vi "APXGauge191119.vi"() -> ()   [LabVIEW 2015]
uses:
  <vilib>/Instr/_visa.llb/VISA Configure Serial Port (Instr).vi
  <userlib>/caLab/Private/Get_PV-1D.vi
  <userlib>/caLab/Private/Put_DBL-1D_PV-1D.vi
  <vilib>/Utility/config.llb/Read Key (String).vi
  <vilib>/Utility/config.llb/NI_LVConfig.lvlib
  <vilib>/Utility/config.llb/Read Key (Path).vi
panel:
  out "APX:SP_SES100":bool
  out "Numeric 3":i32
  in  "stop 2":bool
  out "Numeric 2":i32
  in  "stop":bool
  out "BL132:132WRG1":dbl
  out "SP HIGH":string
  out "SP LOW":string
  out "BL132:SP_BL132":bool
  out "VISA resource name":refnum<visa-resource-name>="COM26"
  out "COM TN908A":refnum<visa-resource-name>="COM10"
  out "APX:GAS":dbl format="%_3f"
  out "APX:AUX":dbl format="%_3f"
  out "COM MAXIGAUGE":refnum<visa-resource-name>
  out "Status":bool
  out "APX:SP_F":bool
  out "APX:SP_E":bool
  out "APX_SP_D":bool
  out "APX:SP_C":bool
  out "APX:SP_B":bool
  out "APX:SP_A":bool
  out "Cycle":i32
  out "APX:HPC001":dbl format="%.6f"
  out "APX:AP2":dbl format="%#_3e"
  out "APX:AP1":dbl format="%#_4g"
  out "APX:PREP":dbl format="%#_3g"
  out "APX:HPC":dbl format="%#_3g"
  out "APX:HPC100":dbl format="%.5g"
  out "APX:SEN6_OFF":bool
  out "APX:SEN6_ON":bool
  out "APX:SEN5_OFF":bool
  out "APX:SEN5_ON":bool
  out "APX:SEN4_OFF":bool
  out "APX:SEN4_ON":bool
  out "APX:SEN3_OFF":bool
  out "APX:SEN3_ON":bool
  out "APX:SEN2_OFF":bool
  out "APX:SEN2_ON":bool
  out "APX:SEN1_OFF":bool
  out "APX:SEN1_ON":bool
  in  "STOP":bool
  # "APX Gauges"
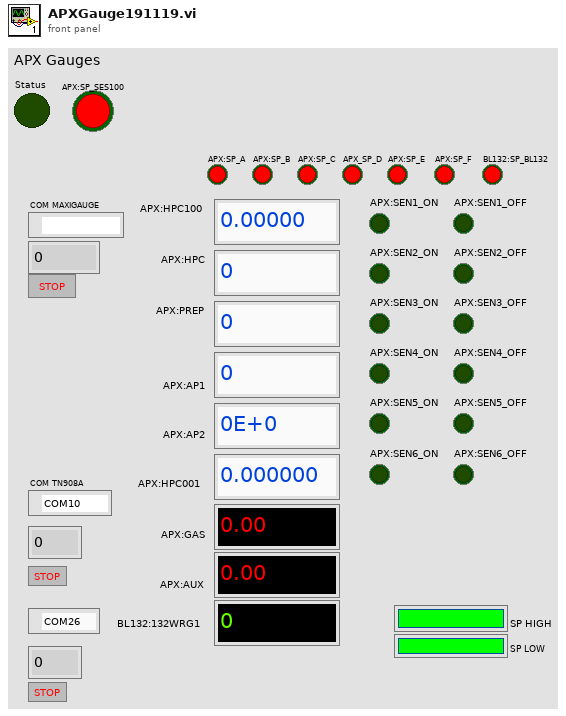
[diagram p1: front panel]
types:
  T1 = typedef "NI_LVConfig.lvlib/Config Data RefNum.ctl" = refnum<k1>
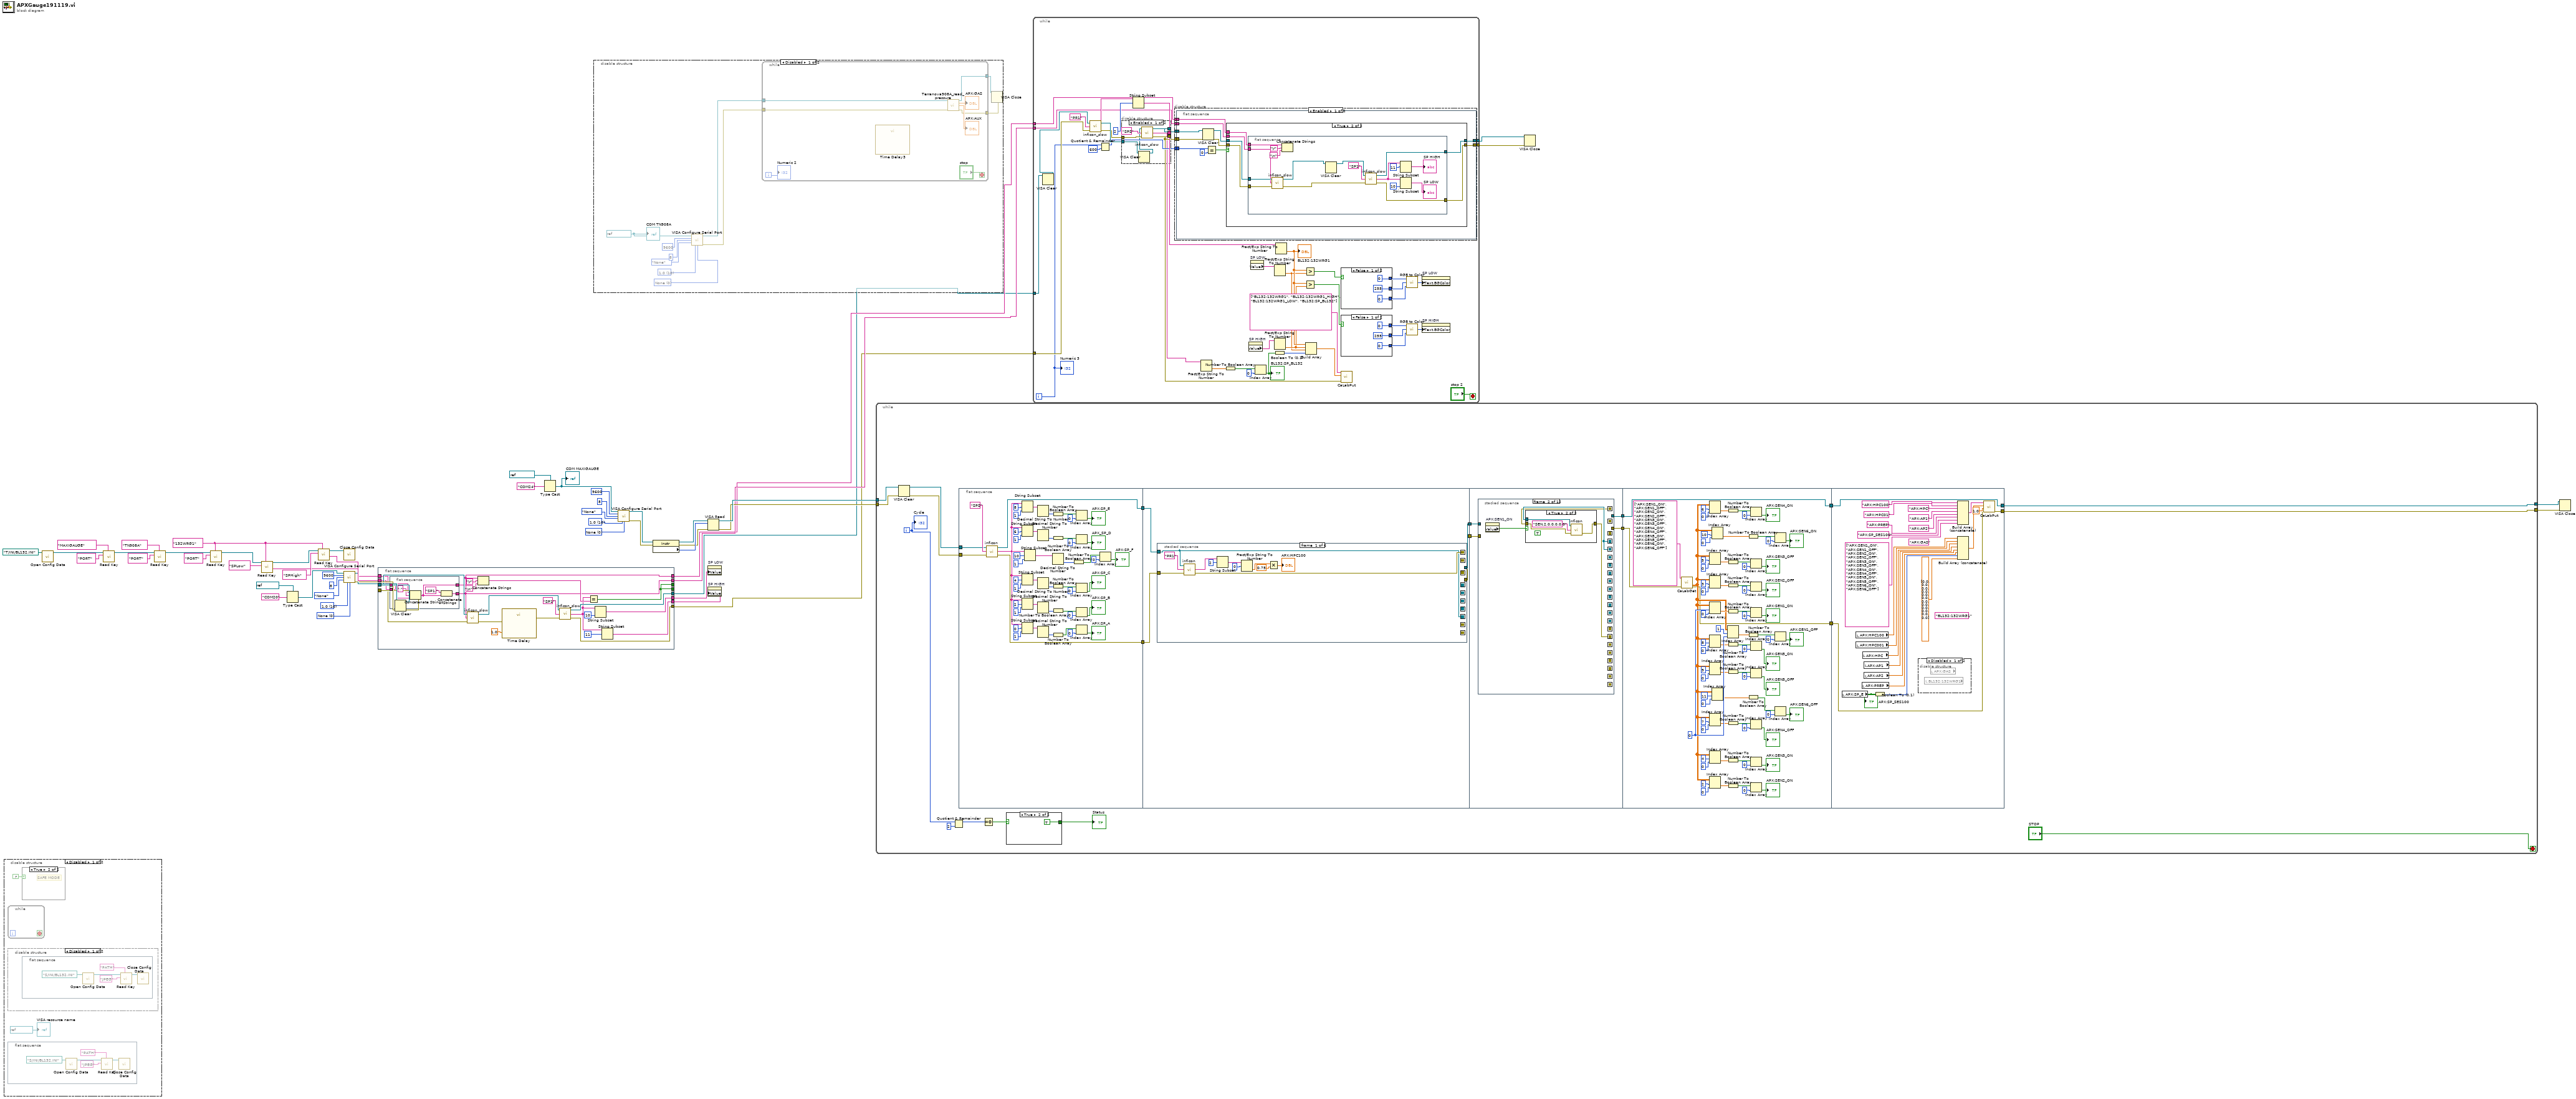
[diagram p0: block diagram]
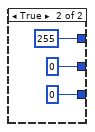
[diagram p6: hidden frame]
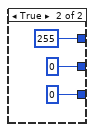
[diagram p7: hidden frame]
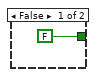
[diagram p11: hidden frame]
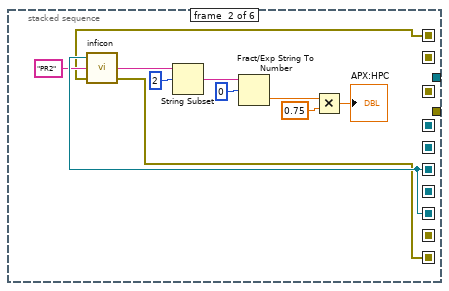
[diagram p12: hidden frame]
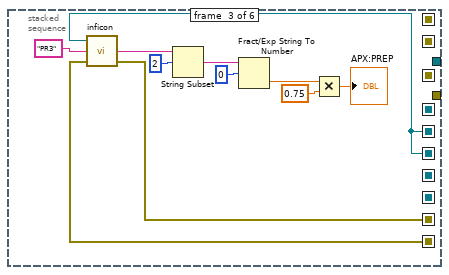
[diagram p13: hidden frame]
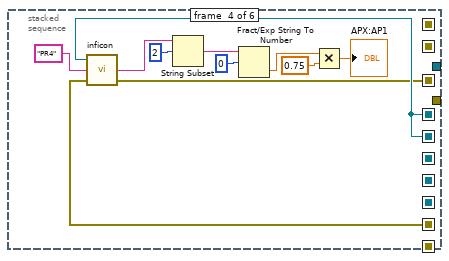
[diagram p14: hidden frame]
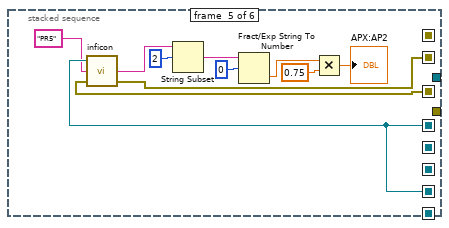
[diagram p15: hidden frame]
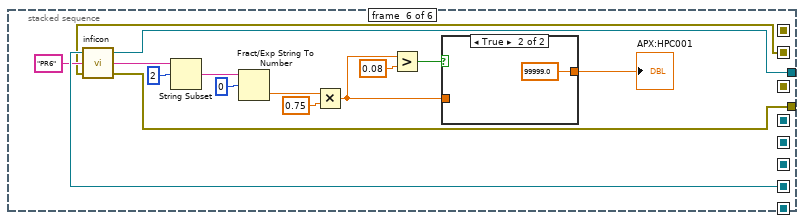
[diagram p16: hidden frame]
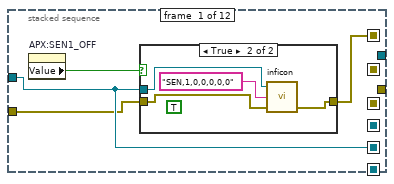
[diagram p18: hidden frame]
diagram:
  w23 = "132WRG1" ("y")
  w33 = u16 10 items=["1.0"=10, "1.5"=15, "2.0"=20] ("stop bits (10: 1 bit)")
  w34 = u16 0 items=["None", "XON/XOFF", "RTS/CTS", "XON/XOFF & RTS/CTS", "DTR/DSR", "XON/XOFF & DTR/DSR"] ("flow control (0:none)")
  w50 = u16 10 items=["1.0"=10, "1.5"=15, "2.0"=20] ("stop bits (10: 1 bit)")
  w51 = u16 0 items=["None", "XON/XOFF", "RTS/CTS", "XON/XOFF & RTS/CTS", "DTR/DSR", "XON/XOFF & DTR/DSR"] ("flow control (0:none)")
  n1 = disable-structure shown="Disabled" {
    frame Disabled {
      n2 = while {
        stop <- _ stop-if-true
      }
      n3 = disable-structure shown="Disabled" {
        frame Disabled {
          n4 = flat-sequence {
            frame #0 {
              n5 = call <vilib>:"Open Config Data.vi"("configuration file path"=path "S:/INI/BL132.INI") -> ("refnum"=w58:T1)  [unwired: 8 in, 2 out]
              n6 = call-poly <vilib>:"Read Key.vi"("section"="PATH" ("key"), "key"="JPEG" ("section"), "refnum"=w58) -> ("value"=w57:path, "refnum out"=w62:T1)  [unwired: 5 in, 2 out]
              n7 = call <vilib>:"Close Config Data.vi"("refnum"=w62) -> ()  [unwired: 9 in, 2 out]
            }
          }
        }
        frame Enabled {
        }
      }
      n8 = flat-sequence {
        frame #0 {
          n9 = call <vilib>:"Open Config Data.vi"("configuration file path"=path "S:/INI/BL132.INI") -> ("refnum"=w63:T1)  [unwired: 8 in, 2 out]
          n10 = call-poly <vilib>:"Read Key.vi"("section"="PATH" ("key"), "key"="JPEG" ("section"), "refnum"=w63) -> ("refnum out"=w67:T1)  [unwired: 5 in, 3 out]
          n11 = call <vilib>:"Close Config Data.vi"("refnum"=w67) -> ()  [unwired: 9 in, 2 out]
        }
      }
      n12 = case shown="True" FALSE {
        frame False {
        }
        frame True {
          # "SAFE MODE"
        }
      }
      "VISA resource name" <- refnum<visa-resource-name> "COM1" ("VISA resource name")
    }
    frame Enabled {
    }
  }
  n13 = call <vilib>:"Open Config Data.vi"("configuration file path"=path "T:/INI/BL132.INI") -> ("refnum"=w12:T1)  [unwired: 8 in, 2 out]
  n14 = call-poly <vilib>:"Read Key.vi"("section"="MAXIGAUGE" ("y"), "key"="PORT" ("y"), "refnum"=w12) -> ("refnum out"=w13:T1)  [unwired: 5 in, 3 out]
  n15 = call-poly <vilib>:"Read Key.vi"("section"="TN908A" ("y"), "key"="PORT" ("y"), "refnum"=w13) -> ("refnum out"=w11:T1)  [unwired: 5 in, 3 out]
  n16 = call-poly <vilib>:"Read Key.vi"("section"=w23, "key"="PORT" ("y"), "refnum"=w11) -> ("refnum out"=w21:T1)  [unwired: 5 in, 3 out]
  n17 = call-poly <vilib>:"Read Key.vi"("section"=w23, "key"="SPLow" ("y"), "refnum"=w21) -> ("value"=w25:string, "refnum out"=w29:T1)  [unwired: 5 in, 2 out]
  n18 = Type Cast(type=refnum<visa-resource-name> "COM1" ("VISA resource name"), x="COM20") -> (*(type *) &x=w31:refnum<visa-resource-name>)
  n19 = call-poly <vilib>:"Read Key.vi"("section"=w23, "key"="SPHigh" ("y"), "refnum"=w29) -> ("value"=w24:string, "refnum out"=w30:T1)  [unwired: 5 in, 2 out]
  n20 = call <vilib>:"Close Config Data.vi"("refnum"=w30) -> ()  [unwired: 9 in, 2 out]
  n21 = call-poly "VISA Configure Serial Port"("VISA resource name"=w31, "baud rate (9600)"=u32 9600, "data bits (8)"=u16 8, "parity (0:none)"=enum16{"None", "Odd", "Even", "Mark", "Space"}."None", "stop bits (10: 1 bit)"=w33, "flow control (0:none)"=w34) -> ("VISA resource name out"=w10:refnum<visa-resource-name>, "error out"=w8:errorcluster)  [unwired: 8 in]
  n22 = flat-sequence {
    tunnel: w9 -> [w86]
    tunnel: w7 -> [w84]
    tunnel: w25 -> [w69]
    tunnel: w24 -> [w68]
    tunnel: [w88] -> w4
    tunnel: [w87] -> w3
    tunnel: [w72] -> _
    tunnel: [w74] -> w18
    tunnel: [w73] -> w19
    tunnel: [w72] -> _
    tunnel: [w71] -> w6
    tunnel: [w70] -> w5
    frame #0 {
      n23 = flat-sequence {
        tunnel: [w92] -> w71
        tunnel: [w93] -> w70
        tunnel: w69 -> [w91]
        tunnel: w68 -> [w90]
        frame #0 {
          n24 = Concatenate Strings(w91, "," ("string to write"), w90) -> (w93:string)
          n25 = Concatenate Strings("SP1," ("string to write"), w93) -> (w92:string)
        }
      }
      n26 = call "inficon_slow.vi"("error out"=w84, "string to write"=w71, "VISA resource name"=w86) -> ("error out 2"=w82:errorcluster, "VISA resource name 2"=w85:refnum<visa-resource-name>)  [unwired: 1 out]
      n27 = Concatenate Strings(w70, "\r", "\n") -> (w80:string)
      n28 = call "Time Delay"("error in (no error)"=w82, "Delay Time (s)"=1.0) -> ("error out"=w83:errorcluster)  [unwired: 9 in]
      n29 = call "inficon_slow.vi"("error out"=w83, "string to write"="SP1", "VISA resource name"=w85) -> ("error out 2"=w87:errorcluster, "read buffer 2"=w76:string, "VISA resource name 2"=w88:refnum<visa-resource-name>)
      n30 = Equal?(x=w76, y=w80) -> (x = y?=w72:bool)
      n31 = String Subset(string=w76, length (rest)=10 ("length (rest)")) -> (substring=w73:string)  [unwired: 1 in]
      n32 = String Subset(string=w76, offset (0)=11) -> (substring=w74:string)  [unwired: 1 in]
    }
  }
  n33 = VISA Clear(VISA resource name=w10, error in (no error)=w8) -> (VISA resource name out=w9:refnum<visa-resource-name>, error out=w7:errorcluster)
  n34 = Type Cast(type=refnum<visa-resource-name> "COM24" ("VISA resource name"), x="COM24") -> (*(type *) &x=w48:refnum<visa-resource-name>)
  "COM MAXIGAUGE" <- w48
  n35 = disable-structure shown="Disabled" {
    frame Disabled {
      w100 = u16 10 items=["1.0"=10, "1.5"=15, "2.0"=20] ("stop bits (10: 1 bit)")
      w101 = u16 0 items=["None", "XON/XOFF", "RTS/CTS", "XON/XOFF & RTS/CTS", "DTR/DSR", "XON/XOFF & DTR/DSR"] ("flow control (0:none)")
      w105 = refnum<visa-resource-name> "COM10" ("VISA resource name")
      n36 = call-poly "VISA Configure Serial Port"("VISA resource name"=w105, "baud rate (9600)"=u32 9600, "data bits (8)"=u16 8, "parity (0:none)"=enum16{"None", "Odd", "Even", "Mark", "Space"}."None", "stop bits (10: 1 bit)"=w100, "flow control (0:none)"=w101) -> ("VISA resource name out"=w99:refnum<visa-resource-name>, "error out"=w98:errorcluster)  [unwired: 8 in]
      n37 = while {
        tunnel: w99 -> [w111]
        tunnel: w98 -> [w110]
        tunnel: [w109] -> w97
        tunnel: [w108] -> w96
        i -> [w106]
        stop <- "stop" stop-if-true
        n38 = call "Time Delay3"() -> ()  [unwired: 11 in, 1 out]
        n39 = call "Terranova908A_read_pressure.vi"("VISA resource name"=w111, "error in (no error)"=w110) -> ("VISA resource name out"=w109:refnum<visa-resource-name>, "pressure"=→"APX:GAS":dbl, "pressure 2"=→"APX:AUX":dbl, "error out"=w108:errorcluster)  [unwired: 9 in, 1 out]
        "Numeric 2" <- w106
      }
      n40 = VISA Close(VISA resource name=w97, error in (no error)=w96) -> ()  [unwired: 1 out]
      "COM TN908A" <- w105
    }
    frame Enabled {
    }
  }
  n41 = call-poly "VISA Configure Serial Port"("VISA resource name"=w48, "baud rate (9600)"=u32 9600, "data bits (8)"=u16 8, "parity (0:none)"=enum16{"None", "Odd", "Even", "Mark", "Space"}."None", "stop bits (10: 1 bit)"=w50, "flow control (0:none)"=w51) -> ("VISA resource name out"=w45:refnum<visa-resource-name>, "error out"=w38:errorcluster)  [unwired: 8 in]
  n42 = property class="Instr"(reference=w45, error in=w38) -> (reference out=w46:refnum<visa-resource-name>, error out=w39:errorcluster, "Serial Settings:Number of Bytes at Serial Port"=w43:u32)
  n43 = VISA Read(VISA resource name=w46, byte count=w43, error in (no error)=w39) -> (VISA resource name out=w44:refnum<visa-resource-name>, error out=w40:errorcluster)  [unwired: 2 out]
  n44 = property on="SP LOW" class="Str"("Value"=w19) -> ()  [unwired: 2 in, 2 out]
  n45 = property on="SP HIGH" class="Str"("Value"=w18) -> ()  [unwired: 2 in, 2 out]
  n46 = while {
    tunnel: [w127] -> w41
    tunnel: w44 -> [w122]
    tunnel: [w130] -> w42
    tunnel: w40 -> [w120]
    i -> [w114]
    stop <- "STOP" stop-if-true
    n47 = VISA Clear(VISA resource name=w122, error in (no error)=w120) -> (VISA resource name out=w121:refnum<visa-resource-name>, error out=w119:errorcluster)
    n48 = Quotient & Remainder(x=w114, y=2) -> (x-y*floor(x/y)=w117:i32)  [unwired: 1 out]
    n49 = flat-sequence {
      tunnel: [w175] -> w132
      tunnel: [w138] -> w126
      tunnel: w121 -> [w137]
      tunnel: w119 -> [w136]
      tunnel: w132 -> [w186]
      tunnel: [w185] -> w131
      tunnel: w126 -> [w187]
      tunnel: [w184] -> w125
      tunnel: w131 -> [w263]
      tunnel: w125 -> [w262]
      tunnel: [w261] -> w124
      tunnel: [w260] -> w123
      tunnel: [w374] -> w129
      tunnel: [w373] -> w128
      tunnel: w124 -> [w372]
      tunnel: w123 -> [w373]
      tunnel: [w470] -> w130
      tunnel: w129 -> [w448]
      tunnel: w128 -> [w470]
      tunnel: [w449] -> w127
      frame #0 {
        n50 = call "inficon.vi"("error out"=w136, "string to write"="SPS", "VISA resource name"=w137) -> ("error out 2"=w138:errorcluster, "read buffer 2"=w144:string, "VISA resource name 2"=w175:refnum<visa-resource-name>)
        n51 = String Subset(string=w144, offset (0)=8, length (rest)=1 ("length (rest)")) -> (substring=w177:string)
        n52 = String Subset(string=w144, offset (0)=6, length (rest)=1 ("length (rest)")) -> (substring=w163:string)
        n53 = String Subset(string=w144, offset (0)=4, length (rest)=1 ("length (rest)")) -> (substring=w169:string)
        n54 = String Subset(string=w144, offset (0)=2, length (rest)=1 ("length (rest)")) -> (substring=w157:string)
        n55 = String Subset(string=w144, offset (0)=0, length (rest)=1 ("length (rest)")) -> (substring=w151:string)
        n56 = String Subset(string=w144, offset (0)=10, length (rest)=1 ("length (rest)")) -> (substring=w145:string)
        n57 = Decimal String To Number(string=w177) -> (number=w178:i32)  [unwired: 2 in, 1 out]
        n58 = Decimal String To Number(string=w163) -> (number=w164:i32)  [unwired: 2 in, 1 out]
        n59 = Decimal String To Number(string=w169) -> (number=w170:i32)  [unwired: 2 in, 1 out]
        n60 = Decimal String To Number(string=w157) -> (number=w158:i32)  [unwired: 2 in, 1 out]
        n61 = Decimal String To Number(string=w151) -> (number=w152:i32)  [unwired: 2 in, 1 out]
        n62 = Decimal String To Number(string=w145) -> (number=w146:i32)  [unwired: 2 in, 1 out]
        n63 = Number To Boolean Array(number=w178) -> (Boolean array=w180:bool[])
        n64 = Number To Boolean Array(number=w164) -> (Boolean array=w166:bool[])
        n65 = Number To Boolean Array(number=w170) -> (Boolean array=w172:bool[])
        n66 = Number To Boolean Array(number=w158) -> (Boolean array=w160:bool[])
        n67 = Number To Boolean Array(number=w152) -> (Boolean array=w154:bool[])
        n68 = Number To Boolean Array(number=w146) -> (Boolean array=w148:bool[])
        n69 = Index Array(array=w180, index=0) -> (element=→"APX:SP_E":bool)
        n70 = Index Array(array=w166, index=0) -> (element=→"APX_SP_D":bool)
        n71 = Index Array(array=w172, index=0) -> (element=→"APX:SP_C":bool)
        n72 = Index Array(array=w160, index=0) -> (element=→"APX:SP_B":bool)
        n73 = Index Array(array=w154, index=0) -> (element=→"APX:SP_A":bool)
        n74 = Index Array(array=w148, index=0) -> (element=→"APX:SP_F":bool)
      }
      frame #1 {
        n75 = stacked-sequence {
          seq-local: [w188 _ _ _ _ _] -> [_ w209 _ _ _ _]
          seq-local: [w190 _ _ _ _ _] -> [_ w200 _ _ _ _]
          seq-local: [_ w209 _ _ _ _] -> [_ _ w220 _ _ _]
          seq-local: [_ w199 _ _ _ _] -> [_ _ w211 _ _ _]
          seq-local: [_ _ w220 _ _ _] -> [_ _ _ w231 _ _]
          seq-local: [_ _ w210 _ _ _] -> [_ _ _ w222 _ _]
          seq-local: [_ _ _ w231 _ _] -> [_ _ _ _ w242 _]
          seq-local: [_ _ _ w221 _ _] -> [_ _ _ _ w232 _]
          seq-local: [_ _ _ _ w242 _] -> [_ _ _ _ _ w257]
          seq-local: [_ _ _ _ w233 _] -> [_ _ _ _ _ w245]
          tunnel: w186 -> [w188 _ _ _ _ _]
          tunnel: w187 -> [w189 _ _ _ _ _]
          tunnel: [_ _ _ _ _ w244] -> w184
          tunnel: [_ _ _ _ _ w243] -> w185
          frame #0 {
            n76 = call "inficon.vi"("error out"=w189, "string to write"="PR1", "VISA resource name"=w188) -> ("error out 2"=w190:errorcluster, "read buffer 2"=w196:string)  [unwired: 1 out]
            n77 = String Subset(string=w196, offset (0)=2) -> (substring=w195:string)  [unwired: 1 in]
            n78 = Fract/Exp String To Number(string=w195, offset=0) -> (number=w191:dbl)  [unwired: 3 out]
            n79 = Multiply(x=w191, y=0.75) -> (x*y=→"APX:HPC100":dbl)
          }
          frame #1 {
            n80 = call "inficon.vi"("error out"=w200, "string to write"="PR2", "VISA resource name"=w209) -> ("error out 2"=w199:errorcluster, "read buffer 2"=w206:string)  [unwired: 1 out]
            n81 = String Subset(string=w206, offset (0)=2) -> (substring=w205:string)  [unwired: 1 in]
            n82 = Fract/Exp String To Number(string=w205, offset=0) -> (number=w201:dbl)  [unwired: 2 in, 1 out]
            n83 = Multiply(x=w201, y=0.75) -> (x*y=→"APX:HPC":dbl)
          }
          frame #2 {
            n84 = call "inficon.vi"("error out"=w211, "string to write"="PR3", "VISA resource name"=w220) -> ("error out 2"=w210:errorcluster, "read buffer 2"=w217:string)  [unwired: 1 out]
            n85 = String Subset(string=w217, offset (0)=2) -> (substring=w215:string)  [unwired: 1 in]
            n86 = Fract/Exp String To Number(string=w215, offset=0 ("offset (0)")) -> (number=w212:dbl)  [unwired: 3 out]
            n87 = Multiply(x=w212, y=0.75) -> (x*y=→"APX:PREP":dbl)
          }
          frame #3 {
            n88 = call "inficon.vi"("error out"=w222, "string to write"="PR4", "VISA resource name"=w231) -> ("error out 2"=w221:errorcluster, "read buffer 2"=w228:string)  [unwired: 1 out]
            n89 = String Subset(string=w228, offset (0)=2) -> (substring=w226:string)  [unwired: 1 in]
            n90 = Fract/Exp String To Number(string=w226, offset=0 ("offset (0)")) -> (number=w223:dbl)  [unwired: 3 out]
            n91 = Multiply(x=w223, y=0.75) -> (x*y=→"APX:AP1":dbl)
          }
          frame #4 {
            n92 = call "inficon.vi"("error out"=w232, "string to write"="PR5", "VISA resource name"=w242) -> ("error out 2"=w233:errorcluster, "read buffer 2"=w239:string)  [unwired: 1 out]
            n93 = String Subset(string=w239, offset (0)=2) -> (substring=w237:string)  [unwired: 1 in]
            n94 = Fract/Exp String To Number(string=w237, offset=0 ("offset (0)")) -> (number=w234:dbl)  [unwired: 3 out]
            n95 = Multiply(x=w234, y=0.75) -> (x*y=→"APX:AP2":dbl)
          }
          frame #5 {
            n96 = call "inficon.vi"("error out"=w245, "string to write"="PR6", "VISA resource name"=w257) -> ("error out 2"=w244:errorcluster, "read buffer 2"=w254:string, "VISA resource name 2"=w243:refnum<visa-resource-name>)
            n97 = String Subset(string=w254, offset (0)=2) -> (substring=w252:string)  [unwired: 1 in]
            n98 = Fract/Exp String To Number(string=w252, offset=0 ("offset (0)")) -> (number=w246:dbl)  [unwired: 3 out]
            n99 = Multiply(x=w246, y=0.75) -> (x*y=w249:dbl)
            n100 = Greater?(x=w249, y=0.08) -> (0:w251:bool)
            n101 = case shown="True" w251 {
              tunnel: w249 -> [w258 _]
              tunnel: [w258 99999.0 ("y")] -> w250
              frame False {
              }
              frame True {
              }
            }
            "APX:HPC001" <- w250
          }
        }
      }
      frame #2 {
        n102 = stacked-sequence {
          seq-local: [w266 _ _ _ _ _ _ _ _ _ _ _] -> [_ w275 _ _ _ _ _ _ _ _ _ _]
          seq-local: [w264 _ _ _ _ _ _ _ _ _ _ _] -> [_ w274 _ _ _ _ _ _ _ _ _ _]
          seq-local: [_ w275 _ _ _ _ _ _ _ _ _ _] -> [_ _ w284 _ _ _ _ _ _ _ _ _]
          seq-local: [_ w273 _ _ _ _ _ _ _ _ _ _] -> [_ _ w283 _ _ _ _ _ _ _ _ _]
          seq-local: [_ _ w284 _ _ _ _ _ _ _ _ _] -> [_ _ _ w293 _ _ _ _ _ _ _ _]
          seq-local: [_ _ w282 _ _ _ _ _ _ _ _ _] -> [_ _ _ w292 _ _ _ _ _ _ _ _]
          seq-local: [_ _ _ w293 _ _ _ _ _ _ _ _] -> [_ _ _ _ w302 _ _ _ _ _ _ _]
          seq-local: [_ _ _ w291 _ _ _ _ _ _ _ _] -> [_ _ _ _ w301 _ _ _ _ _ _ _]
          seq-local: [_ _ _ _ w302 _ _ _ _ _ _ _] -> [_ _ _ _ _ w311 _ _ _ _ _ _]
          seq-local: [_ _ _ _ w300 _ _ _ _ _ _ _] -> [_ _ _ _ _ w310 _ _ _ _ _ _]
          seq-local: [_ _ _ _ _ w311 _ _ _ _ _ _] -> [_ _ _ _ _ _ w320 _ _ _ _ _]
          seq-local: [_ _ _ _ _ w309 _ _ _ _ _ _] -> [_ _ _ _ _ _ w319 _ _ _ _ _]
          seq-local: [_ _ _ _ _ _ w320 _ _ _ _ _] -> [_ _ _ _ _ _ _ w329 _ _ _ _]
          seq-local: [_ _ _ _ _ _ w318 _ _ _ _ _] -> [_ _ _ _ _ _ _ w328 _ _ _ _]
          seq-local: [_ _ _ _ _ _ _ w329 _ _ _ _] -> [_ _ _ _ _ _ _ _ w338 _ _ _]
          seq-local: [_ _ _ _ _ _ _ w327 _ _ _ _] -> [_ _ _ _ _ _ _ _ w337 _ _ _]
          seq-local: [_ _ _ _ _ _ _ _ w338 _ _ _] -> [_ _ _ _ _ _ _ _ _ w347 _ _]
          seq-local: [_ _ _ _ _ _ _ _ w336 _ _ _] -> [_ _ _ _ _ _ _ _ _ w346 _ _]
          seq-local: [_ _ _ _ _ _ _ _ _ w347 _ _] -> [_ _ _ _ _ _ _ _ _ _ w356 _]
          seq-local: [_ _ _ _ _ _ _ _ _ w345 _ _] -> [_ _ _ _ _ _ _ _ _ _ w355 _]
          seq-local: [_ _ _ _ _ _ _ _ _ _ w356 _] -> [_ _ _ _ _ _ _ _ _ _ _ w363]
          seq-local: [_ _ _ _ _ _ _ _ _ _ w354 _] -> [_ _ _ _ _ _ _ _ _ _ _ w365]
          tunnel: w263 -> [w266 _ _ _ _ _ _ _ _ _ _ _]
          tunnel: w262 -> [w265 _ _ _ _ _ _ _ _ _ _ _]
          tunnel: [_ _ _ _ _ _ _ _ _ _ _ w364] -> w261
          tunnel: [_ _ _ _ _ _ _ _ _ _ _ w363] -> w260
          frame #0 {
            n103 = property on="APX:SEN1_OFF" class="Bool (strict)"() -> ("Value"=w267:bool)  [unwired: 2 in, 2 out]
            n104 = case shown="True" w267 {
              tunnel: w266 -> [_ w271]
              tunnel: w265 -> [w268 w270]
              tunnel: [w268 w269] -> w264
              frame False {
              }
              frame True {
                (unwired) TRUE ("Write/Read")
                n105 = call "inficon.vi"("error out"=w270, "string to write"="SEN,1,0,0,0,0,0" ("Command"), "VISA resource name"=w271) -> ("error out 2"=w269:errorcluster)  [unwired: 2 out]
              }
            }
          }
          frame #1 {
            n106 = property on="APX:SEN1_ON" class="Bool (strict)"() -> ("Value"=w276:bool)  [unwired: 2 in, 2 out]
            n107 = case shown="True" w276 {
              tunnel: w275 -> [_ w280]
              tunnel: w274 -> [w277 w279]
              tunnel: [w277 w278] -> w273
              frame False {
              }
              frame True {
                (unwired) TRUE ("Write/Read")
                n108 = call "inficon.vi"("error out"=w279, "string to write"="SEN,2,0,0,0,0,0" ("Command"), "VISA resource name"=w280) -> ("error out 2"=w278:errorcluster)  [unwired: 2 out]
              }
            }
          }
          frame #2 {
            n109 = property on="APX:SEN2_OFF" class="Bool (strict)"() -> ("Value"=w285:bool)  [unwired: 2 in, 2 out]
            n110 = case shown="False" w285 {
              tunnel: w284 -> [_ w289]
              tunnel: w283 -> [w286 w288]
              tunnel: [w286 w287] -> w282
              frame False {
              }
              frame True {
                (unwired) TRUE ("Write/Read")
                n111 = call "inficon.vi"("error out"=w288, "string to write"="SEN,0,1,0,0,0,0" ("Command"), "VISA resource name"=w289) -> ("error out 2"=w287:errorcluster)  [unwired: 2 out]
              }
            }
          }
          frame #3 {
            n112 = property on="APX:SEN2_ON" class="Bool (strict)"() -> ("Value"=w294:bool)  [unwired: 2 in, 2 out]
            n113 = case shown="False" w294 {
              tunnel: w293 -> [_ w298]
              tunnel: w292 -> [w295 w297]
              tunnel: [w295 w296] -> w291
              frame False {
              }
              frame True {
                (unwired) TRUE ("Write/Read")
                n114 = call "inficon.vi"("error out"=w297, "string to write"="SEN,0,2,0,0,0,0" ("Command"), "VISA resource name"=w298) -> ("error out 2"=w296:errorcluster)  [unwired: 2 out]
              }
            }
          }
          frame #4 {
            n115 = property on="APX:SEN3_OFF" class="Bool (strict)"() -> ("Value"=w303:bool)  [unwired: 2 in, 2 out]
            n116 = case shown="False" w303 {
              tunnel: w302 -> [_ w307]
              tunnel: w301 -> [w304 w306]
              tunnel: [w304 w305] -> w300
              frame False {
              }
              frame True {
                (unwired) TRUE ("Write/Read")
                n117 = call "inficon.vi"("error out"=w306, "string to write"="SEN,0,0,1,0,0,0" ("Command"), "VISA resource name"=w307) -> ("error out 2"=w305:errorcluster)  [unwired: 2 out]
              }
            }
          }
          frame #5 {
            n118 = property on="APX:SEN3_ON" class="Bool (strict)"() -> ("Value"=w312:bool)  [unwired: 2 in, 2 out]
            n119 = case shown="False" w312 {
              tunnel: w311 -> [_ w316]
              tunnel: w310 -> [w313 w315]
              tunnel: [w313 w314] -> w309
              frame False {
              }
              frame True {
                (unwired) TRUE ("Write/Read")
                n120 = call "inficon.vi"("error out"=w315, "string to write"="SEN,0,0,2,0,0,0" ("Command"), "VISA resource name"=w316) -> ("error out 2"=w314:errorcluster)  [unwired: 2 out]
              }
            }
          }
          frame #6 {
            n121 = property on="APX:SEN4_OFF" class="Bool (strict)"() -> ("Value"=w321:bool)  [unwired: 2 in, 2 out]
            n122 = case shown="True" w321 {
              tunnel: w320 -> [_ w325]
              tunnel: w319 -> [w322 w324]
              tunnel: [w322 w323] -> w318
              frame False {
              }
              frame True {
                (unwired) TRUE ("Write/Read")
                n123 = call "inficon.vi"("error out"=w324, "string to write"="SEN,0,0,0,1,0,0" ("Command"), "VISA resource name"=w325) -> ("error out 2"=w323:errorcluster)  [unwired: 2 out]
              }
            }
          }
          frame #7 {
            n124 = property on="APX:SEN4_ON" class="Bool (strict)"() -> ("Value"=w330:bool)  [unwired: 2 in, 2 out]
            n125 = case shown="True" w330 {
              tunnel: w329 -> [_ w334]
              tunnel: w328 -> [w331 w333]
              tunnel: [w331 w332] -> w327
              frame False {
              }
              frame True {
                (unwired) TRUE ("Write/Read")
                n126 = call "inficon.vi"("error out"=w333, "string to write"="SEN,0,0,0,2,0,0" ("Command"), "VISA resource name"=w334) -> ("error out 2"=w332:errorcluster)  [unwired: 2 out]
              }
            }
          }
          frame #8 {
            n127 = property on="APX:SEN5_OFF" class="Bool (strict)"() -> ("Value"=w339:bool)  [unwired: 2 in, 2 out]
            n128 = case shown="False" w339 {
              tunnel: w338 -> [_ w343]
              tunnel: w337 -> [w340 w342]
              tunnel: [w340 w341] -> w336
              frame False {
              }
              frame True {
                (unwired) TRUE ("Write/Read")
                n129 = call "inficon.vi"("error out"=w342, "string to write"="SEN,0,0,0,0,1,0" ("Command"), "VISA resource name"=w343) -> ("error out 2"=w341:errorcluster)  [unwired: 2 out]
              }
            }
          }
          frame #9 {
            n130 = property on="APX:SEN5_ON" class="Bool (strict)"() -> ("Value"=w348:bool)  [unwired: 2 in, 2 out]
            n131 = case shown="True" w348 {
              tunnel: w347 -> [_ w352]
              tunnel: w346 -> [w349 w351]
              tunnel: [w349 w350] -> w345
              frame False {
              }
              frame True {
                (unwired) TRUE ("Write/Read")
                n132 = call "inficon.vi"("error out"=w351, "string to write"="SEN,0,0,0,0,2,0" ("Command"), "VISA resource name"=w352) -> ("error out 2"=w350:errorcluster)  [unwired: 2 out]
              }
            }
          }
          frame #10 {
            n133 = property on="APX:SEN6_OFF" class="Bool (strict)"() -> ("Value"=w357:bool)  [unwired: 2 in, 2 out]
            n134 = case shown="False" w357 {
              tunnel: w356 -> [_ w361]
              tunnel: w355 -> [w358 w360]
              tunnel: [w358 w359] -> w354
              frame False {
              }
              frame True {
                (unwired) TRUE ("Write/Read")
                n135 = call "inficon.vi"("error out"=w360, "string to write"="SEN,0,0,0,0,0,1" ("Command"), "VISA resource name"=w361) -> ("error out 2"=w359:errorcluster)  [unwired: 2 out]
              }
            }
          }
          frame #11 {
            n136 = property on="APX:SEN6_ON" class="Bool (strict)"() -> ("Value"=w366:bool)  [unwired: 2 in, 2 out]
            n137 = case shown="True" w366 {
              tunnel: w363 -> [_ w370]
              tunnel: w365 -> [w367 w369]
              tunnel: [w367 w368] -> w364
              frame False {
              }
              frame True {
                (unwired) TRUE ("Write/Read")
                n138 = call "inficon.vi"("error out"=w369, "string to write"="SEN,0,0,0,0,0,2" ("Command"), "VISA resource name"=w370) -> ("error out 2"=w368:errorcluster)  [unwired: 2 out]
              }
            }
          }
        }
      }
      frame #3 {
        w437 = 0 ("index")
        n139 = call-poly "CaLabGet.vi"("PV Names"=string[] ["APX:SEN1_ON", "APX:SEN1_OFF", "APX:SEN2_ON", "APX:SEN2_OFF", "APX:SEN3_ON", "APX:SEN3_OFF", "APX:SEN4_ON", "APX:SEN4_OFF", "APX:SEN5_ON", "APX:SEN5_OFF", "APX:SEN6_ON", "APX:SEN6_OFF"], "Error in (no error)"=w372) -> ("Value Array (number)"=w396:dbl[][], "Error out"=w374:errorcluster)  [unwired: 7 in, 5 out]
        n140 = Index Array(array=w396, index (row)=6 ("disabled index (col)"), index (col)=0) -> (element=w385:dbl)
        n141 = Index Array(array=w396, index (row)=5 ("disabled index (col)"), index (col)=0) -> (element=w387:dbl)
        n142 = Index Array(array=w396, index (row)=3 ("disabled index (col)"), index (col)=0) -> (element=w391:dbl)
        n143 = Index Array(array=w396, index (row)=w437, index (col)=0 ("disabled index (col)")) -> (element=w445:dbl)
        n144 = Index Array(array=w396, index (row)=8 ("disabled index (col)"), index (col)=0) -> (element=w381:dbl)
        n145 = Index Array(array=w396, index (row)=9 ("disabled index (col)"), index (col)=0) -> (element=w379:dbl)
        n146 = Index Array(array=w396, index (row)=7 ("disabled index (col)"), index (col)=0) -> (element=w383:dbl)
        n147 = Index Array(array=w396, index (row)=4 ("disabled index (col)"), index (col)=0) -> (element=w389:dbl)
        n148 = Index Array(array=w396, index (row)=2 ("disabled index (col)"), index (col)=0) -> (element=w393:dbl)
        n149 = Index Array(array=w396, index (row)=10 ("disabled index (col)"), index (col)=0) -> (element=w377:dbl)
        n150 = Index Array(array=w396, index (row)=11 ("disabled index (col)"), index (col)=0) -> (element=w375:dbl)
        n151 = Index Array(array=w396, index (row)=1 ("disabled index (col)"), index (col)=w437) -> (element=w441:dbl)
        n152 = Number To Boolean Array(number=w385) -> (Boolean array=w419:bool[])
        n153 = Number To Boolean Array(number=w387) -> (Boolean array=w423:bool[])
        n154 = Number To Boolean Array(number=w391) -> (Boolean array=w431:bool[])
        n155 = Number To Boolean Array(number=w445) -> (Boolean array=w444:bool[])
        n156 = Number To Boolean Array(number=w381) -> (Boolean array=w411:bool[])
        n157 = Number To Boolean Array(number=w379) -> (Boolean array=w407:bool[])
        n158 = Number To Boolean Array(number=w383) -> (Boolean array=w415:bool[])
        n159 = Number To Boolean Array(number=w389) -> (Boolean array=w427:bool[])
        n160 = Number To Boolean Array(number=w393) -> (Boolean array=w435:bool[])
        n161 = Number To Boolean Array(number=w377) -> (Boolean array=w403:bool[])
        n162 = Number To Boolean Array(number=w441) -> (Boolean array=w440:bool[])
        n163 = Number To Boolean Array(number=w375) -> (Boolean array=w399:bool[])
        n164 = Index Array(array=w419, index=0) -> (element=→"APX:SEN4_ON":bool)
        n165 = Index Array(array=w423, index=0) -> (element=→"APX:SEN3_OFF":bool)
        n166 = Index Array(array=w431, index=0) -> (element=→"APX:SEN2_OFF":bool)
        n167 = Index Array(array=w444, index=0) -> (element=→"APX:SEN1_ON":bool)
        n168 = Index Array(array=w411, index=0) -> (element=→"APX:SEN5_ON":bool)
        n169 = Index Array(array=w407, index=0) -> (element=→"APX:SEN5_OFF":bool)
        n170 = Index Array(array=w415, index=0) -> (element=→"APX:SEN4_OFF":bool)
        n171 = Index Array(array=w427, index=0) -> (element=→"APX:SEN3_ON":bool)
        n172 = Index Array(array=w435, index=0) -> (element=→"APX:SEN2_ON":bool)
        n173 = Index Array(array=w403, index=0) -> (element=→"APX:SEN6_ON":bool)
        n174 = Index Array(array=w440, index=0) -> (element=→"APX:SEN1_OFF":bool)
        n175 = Index Array(array=w399, index=0) -> (element=→"APX:SEN6_OFF":bool)
      }
      frame #4 {
        (unwired) "BL132:132WRG1" ("element")
        (unwired) "APX:GAS"
        n176 = local read "APX:SP_E"() -> (w468:bool)
        "APX:SP_SES100" <- w468
        n177 = local read "APX:HPC100"() -> (w463:dbl)
        n178 = local read "APX:HPC001"() -> (w466:dbl)
        n179 = local read "APX:PREP"() -> (w462:dbl)
        n180 = local read "APX:HPC"() -> (w464:dbl)
        n181 = local read "APX:AP1"() -> (w467:dbl)
        n182 = local read "APX:AP2"() -> (w465:dbl)
        n183 = Boolean To (0,1)(Boolean=w468) -> (0, 1=w469:i16)
        n184 = disable-structure shown="Disabled" {
          frame Disabled {
            n185 = local read "BL132:132WRG1"() -> ()  [unwired: 1 out]
            n186 = local read "APX:GAS"() -> ()  [unwired: 1 out]
          }
          frame Enabled {
          }
        }
        n187 = Build Array (concatenate)("APX:HPC100", "APX:HPC01", "APX:HPC", "APX:AP1", "APX:AP2", "APX:PREP", "APX:SP_SES100" ("element"), string[] ["APX:SEN1_ON", "APX:SEN1_OFF", "APX:SEN2_ON", "APX:SEN2_OFF", "APX:SEN3_ON", "APX:SEN3_OFF", "APX:SEN4_ON", "APX:SEN4_OFF", "APX:SEN5_ON", "APX:SEN5_OFF", "APX:SEN6_ON", "APX:SEN6_OFF"]) -> (w451:string[])
        n188 = Build Array (concatenate)(w463, w466, w464, w467, w465, w462, w469, dbl[] [0.0, 0.0, 0.0, 0.0, 0.0, 0.0, 0.0, 0.0, 0.0, 0.0, 0.0, 0.0]) -> (w450:dbl[])
        n189 = call-poly <userlib>:"CaLabPut.vi"("Error in (no error)"=w448, "Timeout (3)"=1.0, "Values"=w450, "PV Names"=w451) -> ("Error out"=w449:errorcluster)  [unwired: 4 in, 3 out]
      }
    }
    n190 = Equal To 0?(x=w117) -> (x = 0?=w118:bool)
    n191 = case shown="True" w118 {
      tunnel: [FALSE ("Status") TRUE ("Status")] -> w115
      frame False {
      }
      frame True {
      }
    }
    "Status" <- w115
    "Cycle" <- w114
  }
  n192 = while {
    tunnel: w5 -> [w480]
    tunnel: w6 -> [w479]
    tunnel: w4 -> [w473]
    tunnel: w3 -> [w478]
    tunnel: [w475] -> w2
    tunnel: [w474] -> w1
    i -> [w477]
    stop <- "stop 2" stop-if-true
    n193 = VISA Clear(VISA resource name=w473) -> (VISA resource name out=w472:refnum<visa-resource-name>)  [unwired: 1 in, 1 out]
    n194 = call "inficon_slow.vi"("error out"=w478, "string to write"="PR1", "VISA resource name"=w472) -> ("error out 2"=w488:errorcluster, "read buffer 2"=w498:string, "VISA resource name 2"=w512:refnum<visa-resource-name>)
    n195 = Quotient & Remainder(x=w477, y=600) -> (x-y*floor(x/y)=w486:i32)  [unwired: 1 out]
    n196 = disable-structure shown="Enabled" {
      disable-tunnel: [w519 _] -> w485
      disable-tunnel: w488 -> [w518 _]
      disable-tunnel: [w517 _] -> w489
      disable-tunnel: [w516 _] -> w471
      disable-tunnel: w512 -> [w514 _]
      frame Enabled {
        n197 = VISA Clear(VISA resource name=w514) -> (VISA resource name out=w513:refnum<visa-resource-name>)  [unwired: 1 in, 1 out]
        n198 = call "inficon_slow.vi"("error out"=w518, "string to write"="SPS", "VISA resource name"=w513) -> ("error out 2"=w519:errorcluster, "read buffer 2"=w516:string, "VISA resource name 2"=w517:refnum<visa-resource-name>)
      }
      frame Disabled {
      }
    }
    n199 = String Subset(string=w498, offset (0)=2) -> (substring=w496:string)  [unwired: 1 in]
    n200 = disable-structure shown="Enabled" {
      disable-tunnel: w485 -> [w526 _]
      disable-tunnel: w486 -> [w525 _]
      disable-tunnel: w489 -> [w524 _]
      disable-tunnel: w480 -> [w523 _]
      disable-tunnel: w479 -> [w522 _]
      disable-tunnel: [w521 _] -> w475
      disable-tunnel: [w520 _] -> w474
      frame Enabled {
        n201 = flat-sequence {
          tunnel: w523 -> [w535]
          tunnel: w522 -> [w534]
          tunnel: w524 -> [w529]
          tunnel: [w533] -> w520
          tunnel: w526 -> [w530]
          tunnel: [w532] -> w521
          tunnel: w525 -> [w531]
          frame #0 {
            n202 = VISA Clear(VISA resource name=w529, error in (no error)=w530) -> (VISA resource name out=w528:refnum<visa-resource-name>, error out=w527:errorcluster)
            n203 = Equal?(x=w531, y=i16 0) -> (x = y?=w536:bool)
            n204 = case shown="True" w536 {
              tunnel: w535 -> [_ w545]
              tunnel: w534 -> [_ w544]
              tunnel: w528 -> [w538 w543]
              tunnel: w527 -> [w539 w542]
              tunnel: [w539 w541] -> w533
              tunnel: [w538 w540] -> w532
              frame False {
              }
              frame True {
                n205 = flat-sequence {
                  tunnel: w543 -> [w557]
                  tunnel: w542 -> [w556]
                  tunnel: w544 -> [w555]
                  tunnel: w545 -> [w554]
                  tunnel: [w553] -> w541
                  tunnel: [w550] -> w540
                  frame #0 {
                    n206 = call "inficon_slow.vi"("error out"=w556, "string to write"=w555, "VISA resource name"=w557) -> ("error out 2"=w546:errorcluster, "VISA resource name 2"=w549:refnum<visa-resource-name>)  [unwired: 1 out]
                    n207 = Concatenate Strings(w554, "\r", "\n") -> ()  [unwired: 1 out]
                    n208 = VISA Clear(VISA resource name=w549) -> (VISA resource name out=w548:refnum<visa-resource-name>)  [unwired: 1 in, 1 out]
                    n209 = call "inficon_slow.vi"("error out"=w546, "string to write"="SP1", "VISA resource name"=w548) -> ("error out 2"=w553:errorcluster, "read buffer 2"=w547:string, "VISA resource name 2"=w550:refnum<visa-resource-name>)
                    n210 = String Subset(string=w547, offset (0)=11) -> (substring=→"SP HIGH":string)  [unwired: 1 in]
                    n211 = String Subset(string=w547, length (rest)=10 ("length (rest)")) -> (substring=→"SP LOW":string)  [unwired: 1 in]
                  }
                }
              }
            }
          }
        }
      }
      frame Disabled {
      }
    }
    n212 = Fract/Exp String To Number(string=w471) -> (number=w494:dbl)  [unwired: 3 in, 1 out]
    n213 = Number To Boolean Array(number=w494) -> (Boolean array=w493:bool[])
    n214 = property on="SP HIGH" class="Str"() -> ("Value"=w509:string)  [unwired: 2 in, 2 out]
    n215 = property on="SP LOW" class="Str"() -> ("Value"=w510:string)  [unwired: 2 in, 2 out]
    n216 = Index Array(array=w493, index=0) -> (element=w491:bool)
    "BL132:SP_BL132" <- w491
    n217 = Boolean To (0,1)(Boolean=w491) -> (0, 1=w481:i16)
    n218 = Fract/Exp String To Number(string=w510) -> (number=w482:dbl)  [unwired: 3 in, 1 out]
    n219 = Fract/Exp String To Number(string=w509) -> (number=w483:dbl)  [unwired: 3 in, 1 out]
    n220 = Fract/Exp String To Number(string=w496) -> (number=w484:dbl)  [unwired: 3 in, 1 out]
    "BL132:132WRG1" <- w484
    n221 = Greater?(x=w484, y=w482) -> (0:w507:bool)
    n222 = Greater?(x=w484, y=w483) -> (0:w503:bool)
    n223 = Build Array(w484, w483, w482, w481) -> (w495:dbl[])
    n224 = case shown="False" w507 {
      tunnel: [u32 255 ("Text.Text Colors:BG Color") u32 0 ("Text.Text Colors:BG Color")] -> w504
      tunnel: [u32 0 ("Text.Text Colors:BG Color") u32 0 ("Text.Text Colors:BG Color")] -> w505
      tunnel: [u8 0 ("R") u8 255 ("R")] -> w506
      frame False {
      }
      frame True {
      }
    }
    n225 = case shown="False" w503 {
      tunnel: [u32 255 ("Text.Text Colors:BG Color") u32 0 ("Text.Text Colors:BG Color")] -> w499
      tunnel: [u32 0 ("Text.Text Colors:BG Color") u32 0 ("Text.Text Colors:BG Color")] -> w500
      tunnel: [u8 0 ("R") u8 255 ("R")] -> w501
      frame False {
      }
      frame True {
      }
    }
    n226 = call-poly <userlib>:"CaLabPut.vi"("Error in (no error)"=w485, "Values"=w495, "PV Names"=string[] ["BL132:132WRG1", "BL132:132WRG1_HIGH", "BL132:132WRG1_LOW", "BL132:SP_BL132"]) -> ()  [unwired: 5 in, 4 out]
    n227 = call <vilib>:"RGB to Color.vi"("B"=w505, "G"=w504, "R"=w506) -> ("Color"=w508:u32)
    n228 = call <vilib>:"RGB to Color.vi"("B"=w500, "G"=w499, "R"=w501) -> ("Color"=w502:u32)
    n229 = property on="SP LOW" class="Str"("Text.BGColor"=w508) -> ()  [unwired: 2 in, 2 out]
    n230 = property on="SP HIGH" class="Str"("Text.BGColor"=w502) -> ()  [unwired: 2 in, 2 out]
    "Numeric 3" <- w477
  }
  n231 = VISA Close(VISA resource name=w2, error in (no error)=w1) -> ()  [unwired: 1 out]
  n232 = VISA Close(VISA resource name=w42, error in (no error)=w41) -> ()  [unwired: 1 out]
